vi "Obtain Topic From ARN.vi"(8 "error in (no error)":errorcluster, 9 "ARN":string, 10 "Region":T2, 11 "AWS Credentials":T1) -> (0 "error out":errorcluster, 3 "Topic":refnum<class "Topic.lvclass">)   [LabVIEW 2018, in "NI_AWS_SNS.lvlib" / "Topic.lvclass"]
doc: "Alternative constructor for creating a Topic object from a topic ARN"
uses:
  Topic.lvclass
  Core/HTTP Request/Region.ctl
  Core/HTTP Request/AWS Credentials.ctl
  C:/labview-projects/aws-toolkit/source/Core/HTTP Request/HTTP Request.lvclass
  C:/labview-projects/aws-toolkit/source/Core/ARN/ARN.lvclass
  Core/HTTP Request/HTTP Request.lvclass/HTTP Request.ctl
  Core/ARN/ARN.lvclass/ARN.ctl
  Core/HTTP Request/Write Credentials.vi
  Core/HTTP Request/Write Region.vi
  Core/HTTP Request/Write Service.vi
  Core/HTTP Request/Write Verify Server.vi
  Core/ARN/Write ARN.vi
  Core/HTTP Request/HTTP Request.lvclass
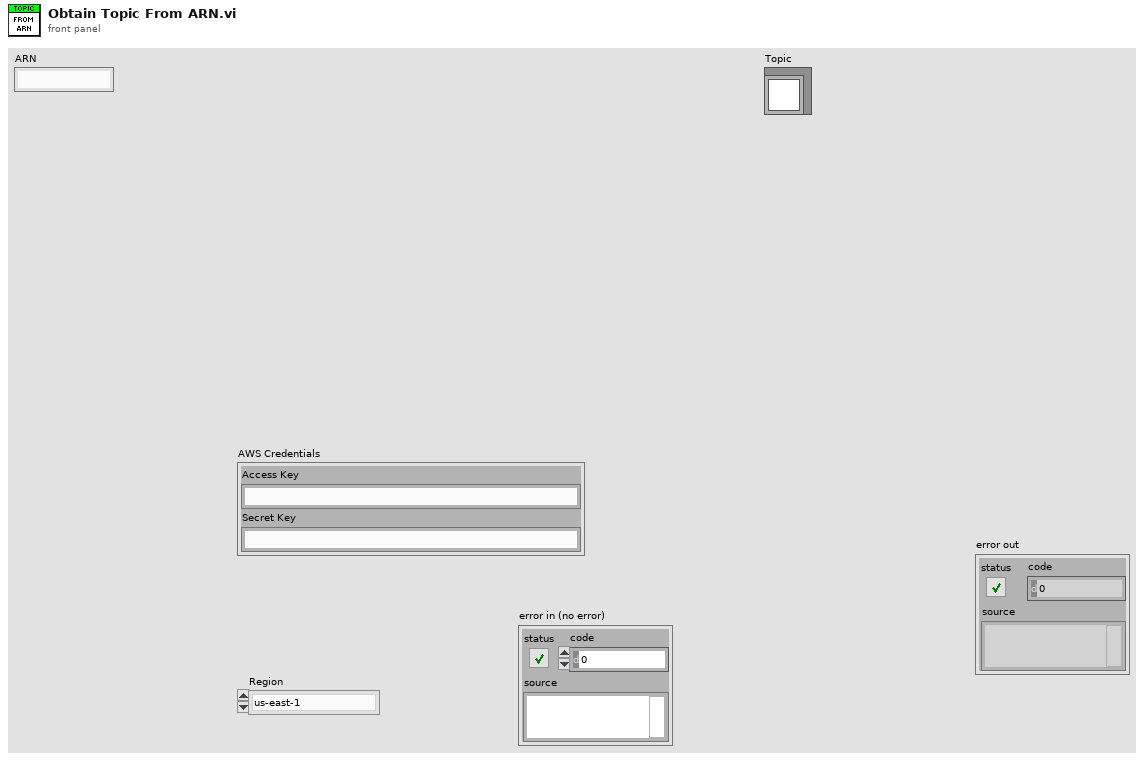
[diagram p1: front panel]
types:
  T1 = typedef "NI_AWS_Core.lvlib/HTTP Request.lvclass/AWS Credentials.ctl" = cluster{"Access Key":string, "Secret Key":string}
  T2 = typedef "NI_AWS_Core.lvlib/HTTP Request.lvclass/Region.ctl" = enum16{"us-east-1", "us-east-2", "us-west-1", "us-west-2", "ap-northeast-1", "ap-northeast-2", "ap-southeast-1", "ap-southeast-2", "ca-central-1", "eu-central-1", "eu-west-1", "eu-west-2", "sa-east-1"}
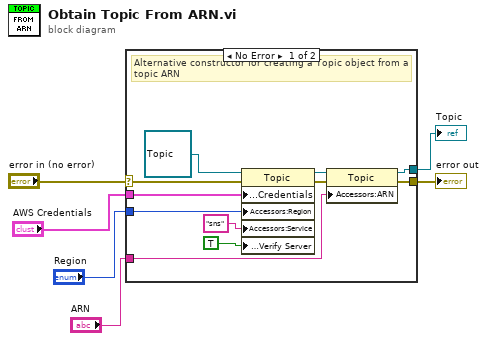
[diagram p0: block diagram]
diagram:
  n1 = case shown="No Error" "error in (no error)" {
    selector: "error in (no error)" -> [w10 w18]
    tunnel: "ARN" -> [w13 _]
    tunnel: "Region" -> [w12 _]
    tunnel: "AWS Credentials" -> [w11 _]
    tunnel: [w8 w18] -> w2
    tunnel: [w7 _] -> w1
    frame No Error {
      # "Alternative constructor for creating a Topic object from a topic ARN"
      n2 = property class="Topic"(reference=refnum<class "Topic.lvclass"> refnum ("NI_AWS_SNS.lvlib:Topic"), error in=w10, "Accessors:Credentials"=w11, "Accessors:Region"=w12, "Accessors:Service"="sns" ("Service"), "Accessors:Verify Server"=TRUE ("Verify Server")) -> (reference out=w14:refnum<class "Topic.lvclass">, error out=w9:errorcluster)
      n3 = property class="Topic"(reference=w14, error in=w9, "Accessors:ARN"=w13) -> (reference out=w7:refnum<class "Topic.lvclass">, error out=w8:errorcluster)
    }
    frame Error {
    }
  }
  "error out" <- w2
  "Topic" <- w1
